vi "Treat Data Name.vi"(8 "error in (no error)":errorcluster, 11 "Data":variant) -> (0 "error out":errorcluster, 1 "untreated Data Name":string, 2 "EasyXML Type":T1, 3 "dup Data":variant, 4 "contains raw xml?":bool, 5 "treated xml name":string, 7 "attributes cluster?":bool)   [LabVIEW 2013]
uses:
  Type Defs/Formatting Data Type -- Enum.ctl
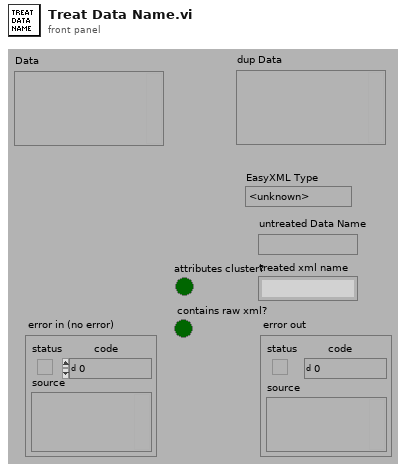
[diagram p1: front panel]
types:
  T1 = typedef "Formatting Data Type -- Enum.ctl" = enum16{"<unknown>", "Cluster", "Array", "String", "Path", "Boolean", "Time Stamp", "Enum", "Numeric - EXT", "Numeric - DBL", "Numeric - SGL", "Numeric - I64", "Numeric - I32", "Numeric - I16", "Numeric - I8", "Numeric - U64", "Numeric - U32", "Numeric - U16", "Numeric - U8", "Numeric - CXT", "Numeric - CDB", "Numeric - CSG", "VISA Resource"}
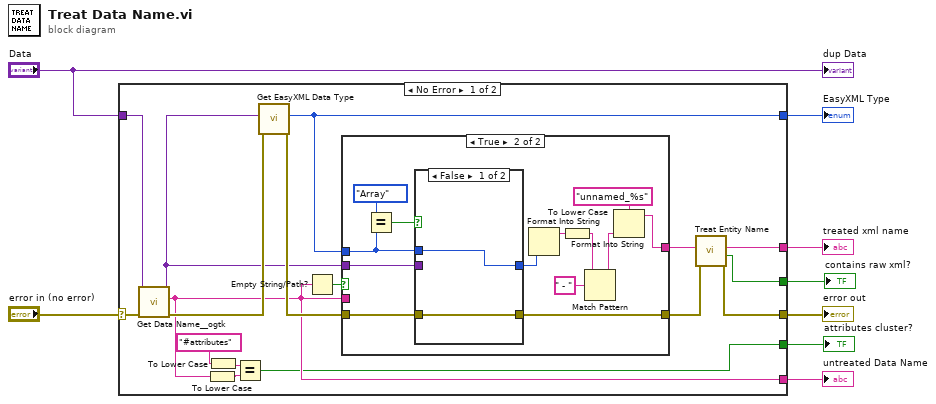
[diagram p0: block diagram]
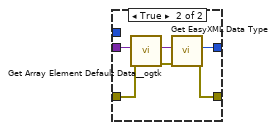
[diagram p3: hidden frame]
diagram:
  n1 = case shown="No Error" "error in (no error)" {
    selector: "error in (no error)" -> [w25 w49]
    tunnel: [w19 _] -> w8
    tunnel: [w17 w49] -> w6
    tunnel: "Data" -> [w24 _]
    tunnel: [w20 _] -> w5
    tunnel: [w10 _] -> w3
    tunnel: [w14 _] -> w2
    tunnel: [w9 _] -> w1
    frame No Error {
      n2 = call <userlib>:"Get Data Name__ogtk.vi"("error in (no error)"=w25, "Data"=w24) -> ("error out"=w23:errorcluster, "Data Name"=w10:string, "Data dup"=w15:variant)  [unwired: 7 in]
      n3 = To Lower Case(string=w10) -> (all lower case string=w11:string)
      n4 = To Lower Case(string="#attributes" ("Data Name")) -> (all lower case string=w12:string)
      n5 = Equal?(x=w12, y=w11) -> (x = y?=w9:bool)
      n6 = call "Get EasyXML Data Type.vi"("error in"=w23, "LabVIEW Data"=w15) -> ("error out"=w22:errorcluster, "EasyXML Type"=w20:T1)  [unwired: 8 in]
      n7 = Empty String/Path?(string/path=w10) -> (empty?=w21:bool)
      n8 = case shown="True" w21 {
        tunnel: w20 -> [_ w31]
        tunnel: w22 -> [w27 w34]
        tunnel: [w27 w33] -> w16
        tunnel: w10 -> [w26 _]
        tunnel: [w26 w38] -> w18
        tunnel: w15 -> [_ w35]
        frame False {
        }
        frame True {
          n9 = Equal?(x=Formatting_Data_Type_--_Enum."Array", y=w31) -> (x = y?=w36:bool)
          n10 = case shown="False" w36 {
            tunnel: w35 -> [_ w48]
            tunnel: w34 -> [w41 w47]
            tunnel: [w41 w44] -> w33
            tunnel: [w42 w43] -> w32
            tunnel: w31 -> [w42 _]
            frame False {
            }
            frame True {
              n11 = call <userlib>:"Get Array Element Default Data__ogtk.vi"("error in (no error)"=w47, "Array"=w48) -> ("error out"=w45:errorcluster, "Array Element Default Data"=w46:variant)  [unwired: 8 in]
              n12 = call "Get EasyXML Data Type.vi"("error in"=w45, "LabVIEW Data"=w46) -> ("error out"=w44:errorcluster, "EasyXML Type"=w43:T1)  [unwired: 8 in]
            }
          }
          n13 = Format Into String(w32) -> (resulting string=w39:string)  [unwired: 3 in, 1 out]
          n14 = To Lower Case(string=w39) -> (all lower case string=w28:string)
          n15 = Match Pattern(string=w28, regular expression=" - ") -> (before substring=w29:string)  [unwired: 1 in, 3 out]
          n16 = Format Into String(format string="unnamed_%s" ("string"), w29) -> (resulting string=w38:string)  [unwired: 2 in, 1 out]
        }
      }
      n17 = call "Treat Entity Name.vi"("error in"=w16, "Data Name"=w18) -> ("error out"=w17:errorcluster, "contains raw xml?"=w14:bool, "Entity Name"=w19:string)  [unwired: 7 in]
    }
    frame Error {
    }
  }
  "treated xml name" <- w8
  "EasyXML Type" <- w5
  "error out" <- w6
  "untreated Data Name" <- w3
  "contains raw xml?" <- w2
  "attributes cluster?" <- w1
  "dup Data" <- "Data"
